vi "Corriente_vrms.vi"(11 "Dynamic Data":dynamicdata(waveform)) -> (1 "Scalar":dbl, 2 "Boolean":bool, 3 "Waveform":waveform(dbl))   [LabVIEW 2019]
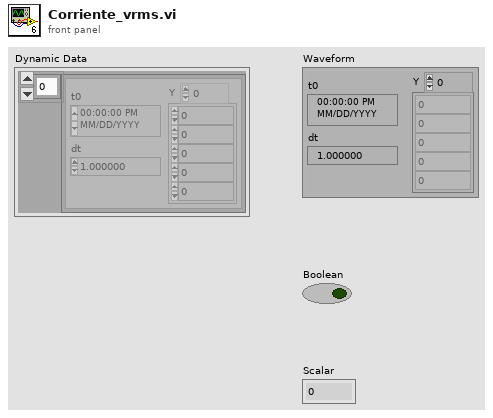
[diagram p1: front panel]
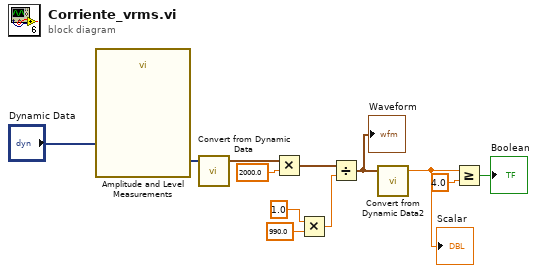
[diagram p0: block diagram]
diagram:
  n1 = call "Amplitude and Level Measurements"("Signals"="Dynamic Data") -> ("RMS"=w2:dynamicdata)  [unwired: 13 in, 1 out]
  n2 = call "Convert from Dynamic Data"("Dynamic Data Type"=w2) -> ("Waveform"=w3:waveform(dbl))  [unwired: 3 in]
  n3 = Multiply(x=w3, y=2000.0) -> (x*y=w6:waveform(dbl))
  n4 = Multiply(x=1.0, y=990.0) -> (x*y=w7:dbl)
  n5 = Divide(x=w6, y=w7) -> (x/y=w8:waveform(dbl))
  "Waveform" <- w8
  n6 = call "Convert from Dynamic Data2"("Dynamic Data Type"=w8) -> ("Scalar"=w9:dbl)  [unwired: 3 in]
  "Scalar" <- w9
  n7 = Greater Or Equal?(x=w9, y=4.0) -> (x >= y?=→"Boolean":bool)
